vi "UserCommentToVersion.vi"(11 "User Comment":string) -> (2 "BlueSerializableVersion found?":bool, 3 "BlueSerializableVersion":u16)   [LabVIEW 2019, in "BlueSerializationProviderShared.lvlib"]
uses:
  BlueSerializationProviderShared.lvlib
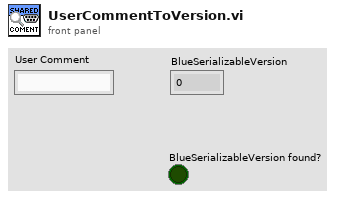
[diagram p1: front panel]
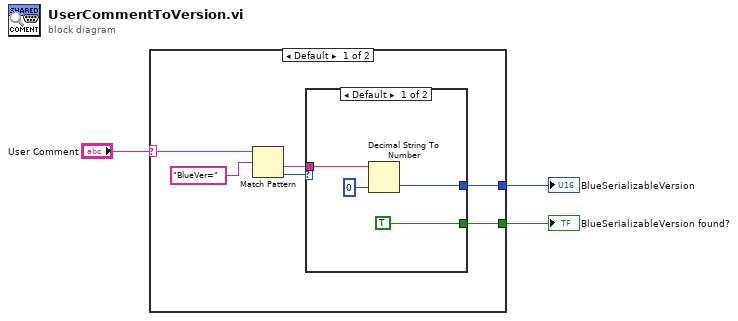
[diagram p0: block diagram]
diagram:
  n1 = case shown="Default" "User Comment" {
    selector: "User Comment" -> [w8 _]
    tunnel: [w5 _] -> w1
    tunnel: [w4 _] -> w2
    frame Default {
      n2 = Match Pattern(string=w8, regular expression="BlueVer=") -> (after substring=w6:string, offset past match=w7:i32)  [unwired: 1 in, 2 out]
      n3 = case shown="Default" w7 {
        tunnel: w6 -> [w13 _]
        tunnel: [TRUE _] -> w5
        tunnel: [w10 _] -> w4
        frame Default {
          n4 = Decimal String To Number(string=w13, default (0L)=u16 0 ("default (0 I32)")) -> (number=w10:u16)  [unwired: 1 in, 1 out]
        }
        frame -1 {
        }
      }
    }
    frame "" {
    }
  }
  "BlueSerializableVersion" <- w2
  "BlueSerializableVersion found?" <- w1
